vi "Best_Fit_FOAW.vi"(0 "y_k":dbl, 1 "d":dbl, 2 "T":dbl, 3 "n_max":i32=10, 4 "Initialize":bool) -> (7 "vel estimation":dbl, 9 "window length":i32)   [LabVIEW 2019]
panel:
  in  "found":bool
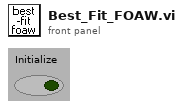
[diagram p1: front panel]
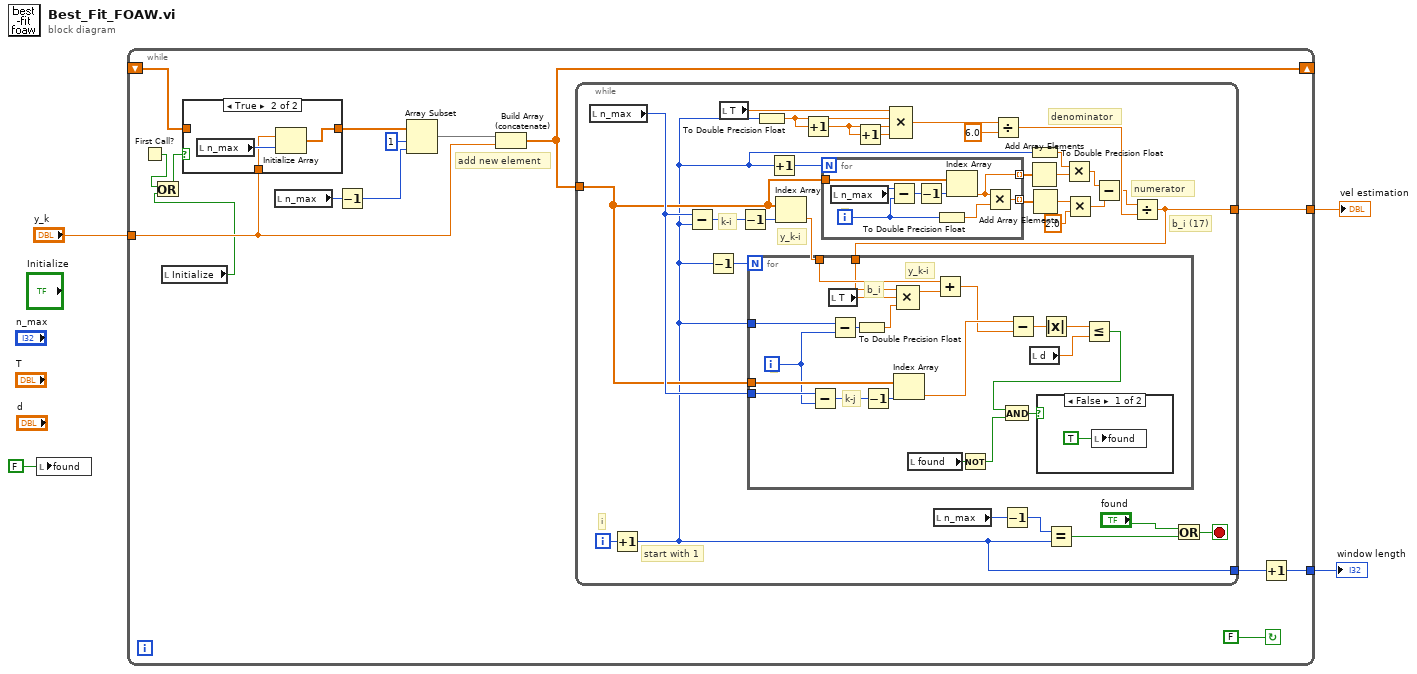
[diagram p0: block diagram]
diagram:
  n1 = local write "found"(FALSE ("found")) -> ()
  n2 = while {
    tunnel: "y_k" -> [w8]
    tunnel: [w18] -> w2
    shift-right: [w12] -> _
    shift-left: _ -> [w13]
    tunnel: [w10] -> w1
    stop <- FALSE continue-if-true
    # "add new element"
    n3 = First Call?() -> (First Call?: T/F=w7:bool)
    n4 = local read "Initialize"() -> (w5:bool)
    n5 = Or(x=w7, y=w5) -> (x .or. y?=w6:bool)
    n6 = case shown="True" w6 {
      tunnel: [w20 w22] -> w9
      tunnel: w13 -> [w20 _]
      tunnel: w8 -> [_ w21]
      frame False {
      }
      frame True {
        n7 = local read "n_max"() -> (w23:i32)
        n8 = Initialize Array(w21, w23) -> (w22:dbl[])
      }
    }
    n9 = local read "n_max"() -> (w16:i32)
    n10 = Decrement(x=w16) -> (x-1=w15:i32)
    n11 = Array Subset(array=w9, index=1, length=w15) -> (w14:dbl[])
    n12 = Build Array (concatenate)(w14, w8) -> (w12:dbl[])
    n13 = while {
      tunnel: w12 -> [w35]
      tunnel: [w46] -> w18
      tunnel: [w31] -> w11
      i -> [w49]
      stop <- w52 stop-if-true
      # "numerator"
      # "b_i (17)"
      # "i"
      # "start with 1"
      # "y_k-i"
      # "denominator"
      # "k-i"
      n14 = local read "n_max"() -> (w47:i32)
      n15 = Increment(x=w49) -> (x+1=w31:i32)
      n16 = Subtract(x=w47, y=w31) -> (x-y=w54:i32)
      n17 = Decrement(x=w31) -> (x-1=w48:i32)
      n18 = local read "T"() -> (w44:dbl)
      n19 = Decrement(x=w54) -> (x-1=w37:i32)
      n20 = To Double Precision Float(number=w31) -> (double precision float=w43:dbl)
      n21 = Increment(x=w31) -> (x+1=w25:i32)
      n22 = Index Array(array=w35, index=w37) -> (element=w38:dbl)
      n23 = Increment(x=w43) -> (x+1=w42:dbl)
      n24 = for {
        N: w25 -> [_]
        tunnel: w35 -> [w62]
        tunnel: [w60] -> w34 mode=indexing
        tunnel: [w59] -> w33 mode=indexing
        i -> [w57]
        # "j"
        n25 = local read "n_max"() -> (w58:i32)
        n26 = Subtract(x=w58, y=w57) -> (x-y=w56:i32)
        n27 = Decrement(x=w56) -> (x-1=w55:i32)
        n28 = To Double Precision Float(number=w57) -> (double precision float=w61:dbl)
        n29 = Index Array(array=w62, index=w55) -> (element=w59:dbl)
        n30 = Multiply(x=w59, y=w61) -> (x*y=w60:dbl)
      }
      n31 = Increment(x=w42) -> (x+1=w41:dbl)
      n32 = Compound Arithmetic op=MULTIPLY(w44, w43, w42, w41) -> (w24:dbl)
      n33 = local read "n_max"() -> (w51:i32)
      n34 = Divide(x=w24, y=6.0) -> (x/y=w40:dbl)
      n35 = Decrement(x=w51) -> (x-1=w45:i32)
      n36 = Add Array Elements(numeric array=w33) -> (sum=w32:dbl)
      n37 = To Double Precision Float(number=w31) -> (double precision float=w30:dbl)
      n38 = Add Array Elements(numeric array=w34) -> (sum=w36:dbl)
      n39 = Equal?(x=w45, y=w31) -> (x = y?=w50:bool)
      n40 = Multiply(x=w30, y=w32) -> (x*y=w27:dbl)
      n41 = Multiply(x=w36, y=2.0) -> (x*y=w28:dbl)
      n42 = Subtract(x=w27, y=w28) -> (x-y=w26:dbl)
      n43 = Divide(x=w26, y=w40) -> (x/y=w46:dbl)
      n44 = for {
        N: w48 -> [_]
        tunnel: w35 -> [w73]
        tunnel: w38 -> [w80]
        tunnel: w46 -> [w77]
        tunnel: w31 -> [w76]
        tunnel: w47 -> [w71]
        i -> [w70]
        # "b_i"
        # "y_k-i"
        # "k-j"
        # "j"
        n45 = Subtract(x=w71, y=w70) -> (x-y=w72:i32)
        n46 = local read "T"() -> (w78:dbl)
        n47 = Subtract(x=w76, y=w70) -> (x-y=w75:i32)
        n48 = To Double Precision Float(number=w75) -> (double precision float=w74:dbl)
        n49 = Decrement(x=w72) -> (x-1=w63:i32)
        n50 = Index Array(array=w73, index=w63) -> (element=w69:dbl)
        n51 = Compound Arithmetic op=MULTIPLY(w77, w78, w74) -> (w79:dbl)
        n52 = local read "found"() -> (w82:bool)
        n53 = Add(x=w80, y=w79) -> (x+y=w68:dbl)
        n54 = Not(x=w82) -> (.not. x?=w81:bool)
        n55 = Subtract(x=w69, y=w68) -> (x-y=w67:dbl)
        n56 = local read "d"() -> (w65:dbl)
        n57 = Absolute Value(x=w67) -> (abs(x)=w66:dbl)
        n58 = Less Or Equal?(x=w66, y=w65) -> (x <= y?=w64:bool)
        n59 = And(x=w64, y=w81) -> (x .and. y?=w83:bool)
        n60 = case shown="False" w83 {
          frame False {
            n61 = local write "found"(TRUE ("found")) -> ()
          }
          frame True {
          }
        }
      }
      n62 = Or(x="found", y=w50) -> (x .or. y?=w52:bool)
    }
    n63 = Increment(x=w11) -> (x+1=w10:i32)
  }
  "vel estimation" <- w2
  "window length" <- w1
